vi "Get DSF Configuration Runtime File Path.vi"(8 "error in (no error)":errorcluster, 11 "Item Ref in":T1 format="%.0x") -> (0 "error out":errorcluster, 1 "Found":bool, 2 "Path":path, 3 "Item Ref out":T1 format="%.0x")   [LabVIEW 2017, in "Data Sharing Framework Engine.lvlib"]
uses:
  <vilib>/NI Veristand/Custom Device API/Custom Device Item Ref.ctl
  <vilib>/NI Veristand/Custom Device API/Custom Device Target Type.ctl
  <vilib>/NI Veristand/Custom Device API/Get Item Property (Dependent File).vi
  Data Sharing Framework Engine.lvlib
  <vilib>/NI Veristand/Custom Device API/Custom Device API.lvlib
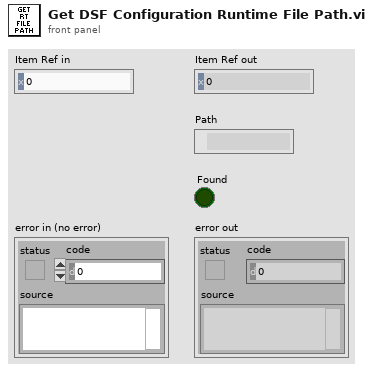
[diagram p1: front panel]
types:
  T1 = typedef "Custom Device API.lvlib/Custom Device Item Ref.ctl" = u64
  T2 = typedef "Custom Device API.lvlib/Custom Device Target Type.ctl" = enum16{"PharLap", "VxWorks", "Windows", "Linux_32_ARM", "Linux_x64"}
  T3 = typedef "Custom Device API.lvlib/Dependent File Optional Info.ctl" = cluster{"Version":string, "RTDestination":path, "ForceDownload":bool, "SupportedTarget":string, "MD5":string}
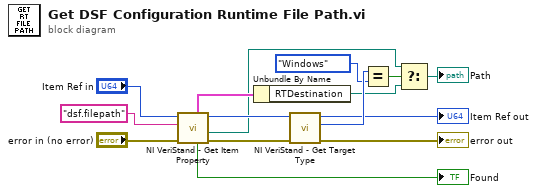
[diagram p0: block diagram]
diagram:
  n1 = call-poly <vilib>:"NI VeriStand - Get Item Property.vi"("error in (no error)"="error in (no error)", "Property Name"="dsf.filepath", "Item Ref in"="Item Ref in") -> ("error out"=w3:errorcluster, "Path"=w9:path, "Item Ref out"=w13:T1, "Found"=→"Found":bool, "OptionalInfo"=w14:T3)  [unwired: 4 in]
  n2 = Unbundle By Name(w14) -> ("RTDestination"=w8:path)
  n3 = call <vilib>:"NI VeriStand - Get Target Type.vi"("error in (no error)"=w3, "Item Ref in"=w13) -> ("error out"=→"error out":errorcluster, "Target Type"=w12:T2, "Item Ref out"=→"Item Ref out":T1)  [unwired: 7 in]
  n4 = Equal?(x=w12, y=Custom_Device_Target_Type."Windows") -> (x = y?=w10:bool)
  n5 = Select(t=w9, s=w10, f=w8) -> (s? t:f=→"Path":path)
